vi "CalibrateGyro.vi"   [LabVIEW 2016, in "LEGO-PMR.lvrbt"]
uses:
  LEGO-PMR.lvrbt
  <vilib>/NXT/Block Support/NXT_InputPort.ctl
  <vilib>/NXT/Dual Mode Library/Waits/Wait_Num.vi
  <vilib>/NXT/Dual Mode Library/Sensors/EV3_Gyro_Angle.vi
  <vilib>/NXT/Dual Mode Library/Sensors/EV3_Gyro_Rate.vi
types:
  T1 = typedef "NXT_InputPort.ctl" = u32
  T2 = typedef "LVHSConnector.ctl" = refnum<class "BrickReference.lvclass">
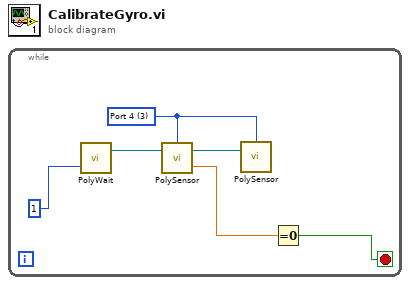
[diagram p0: block diagram]
diagram:
  n1 = while {
    stop <- w1 stop-if-true
    w3 = T1 3 items=["Port 1", "Port 2", "Port 3", "Port 4"] ("Port (Port 1)")
    n2 = call-poly <vilib>:"PolyWait.vi"("Time (1 sec)"=1) -> ("NXT/EV3"=w5:T2)  [unwired: 3 in]
    n3 = call-poly <vilib>:"PolySensor.vi"("NXT/EV3"=w5, "Port (Port 1)"=w3) -> ("Degrees"=w2:sgl, "NXT/EV3"=w4:T2)  [unwired: 1 in]
    n4 = call-poly <vilib>:"PolySensor.vi"("NXT/EV3"=w4, "Port (Port 1)"=w3) -> ()  [unwired: 1 in, 2 out]
    n5 = Equal To 0?(x=w2) -> (x = 0?=w1:bool)
  }
